vi "Relativize Paths.vi"(10 "Valid File Paths":path[](array[path]), 11 "Target Folder":path) -> (3 "Array":string[](array[string]))   [LabVIEW 2019, in "AutoMenuCreator.lvlib"]
uses:
  AutoMenuCreator.lvlib
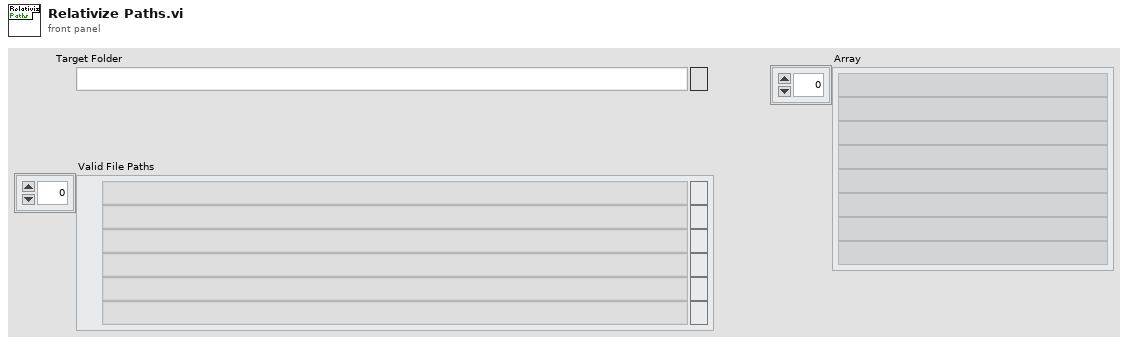
[diagram p1: front panel]
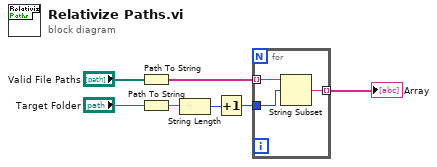
[diagram p0: block diagram]
diagram:
  n1 = Path To String(path="Valid File Paths") -> (string=w3:string[])
  n2 = Path To String(path="Target Folder") -> (string=w4:string)
  n3 = String Length(string=w4) -> (length=w2:i32)
  n4 = Increment(x=w2) -> (x+1=w1:i32)
  n5 = for {
    tunnel: w3 -> [w10] mode=indexing
    tunnel: w1 -> [w9]
    tunnel: [w8] -> w7 mode=indexing
    n6 = String Subset(string=w10, offset (0)=w9) -> (substring=w8:string)  [unwired: 1 in]
  }
  "Array" <- w7
